vi "Read Current Command Code.vi"(8 "error in (no error)":errorcluster, 11 "AK TCP in":refnum<class "AK TCP.lvclass">) -> (0 "error out":errorcluster, 2 "Current Command Code":string, 3 "AK TCP out":refnum<class "AK TCP.lvclass">)   [LabVIEW 2019, in "Protocols.lvlib" / "AK TCP.lvclass"]
uses:
  AK TCP.lvclass
  AK TCP.lvclass/AK TCP.ctl
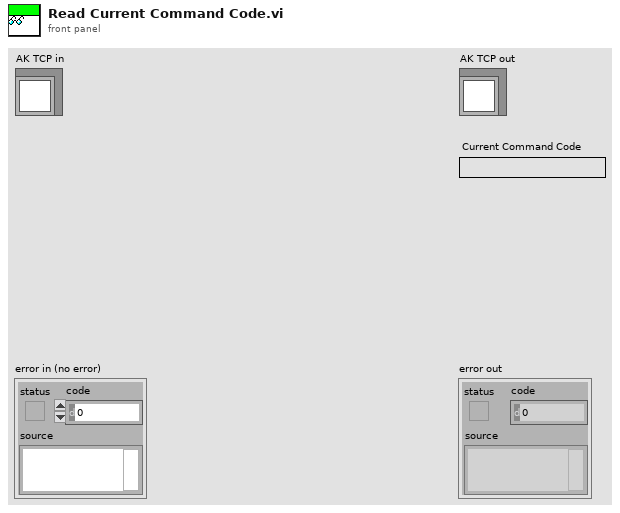
[diagram p1: front panel]
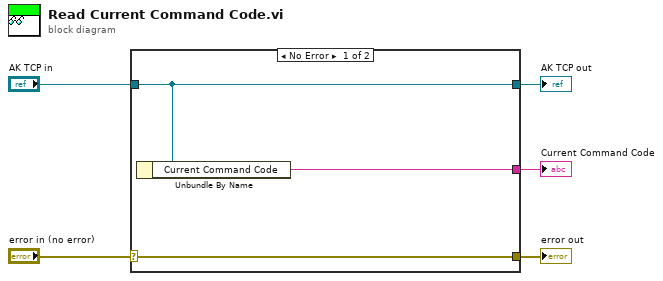
[diagram p0: block diagram]
diagram:
  n1 = case shown="No Error" "error in (no error)" {
    selector: "error in (no error)" -> [w8 w9]
    tunnel: [w8 w9] -> w4
    tunnel: [w7 w10] -> w2
    tunnel: "AK TCP in" -> [w7 w10]
    tunnel: [w6 _] -> w1
    frame No Error {
      n2 = Unbundle By Name(w7) -> ("Current Command Code"=w6:string)
    }
    frame Error {
    }
  }
  "error out" <- w4
  "AK TCP out" <- w2
  "Current Command Code" <- w1
